vi "Update Mock Class.vi"(8 "error in (no error)":errorcluster, 10 "Mock Class Path":path=path "C:/Users/AntonSundqvist/Desktop/New folder/test.lvclass") -> (0 "error out":errorcluster)   [LabVIEW 2020, in "Mock Class Updater.lvclass"]
uses:
  Mock Class Updater.lvclass
  Mock Class Updater.lvclass/Mock Class Updater.ctl
  Mock Class Generator/Mock Class Generator.lvclass
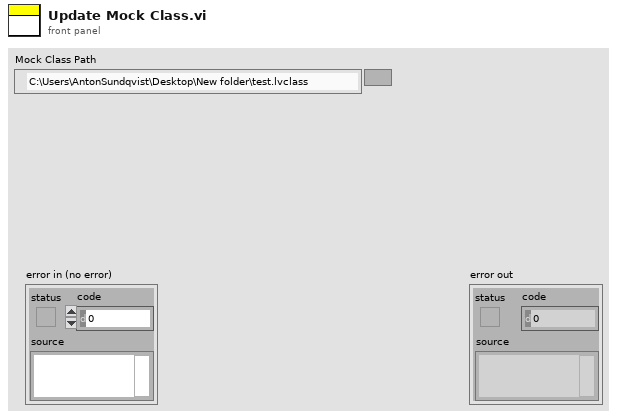
[diagram p1: front panel]
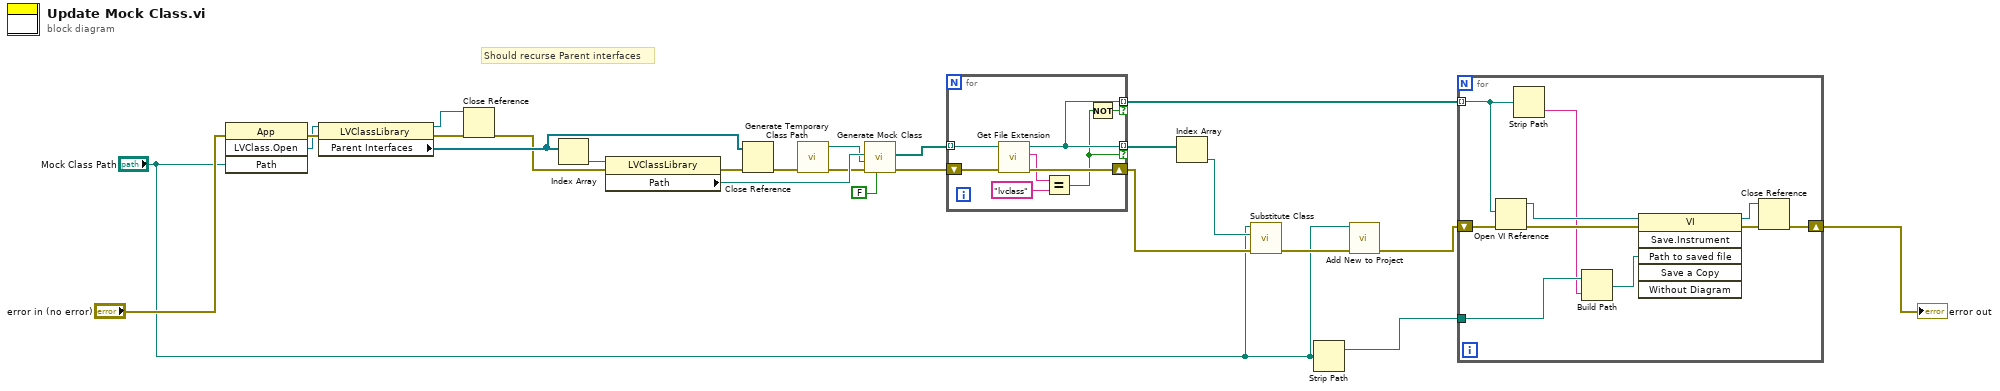
[diagram p0: block diagram]
diagram:
  # "Should recurse Parent interfaces"
  n1 = invoke class="App" method="LVClass.Open"(error in="error in (no error)", "Path"="Mock Class Path") -> (error out=w24:errorcluster, "LVClass.Open"=w23:refnum<vi>)  [unwired: 2 in, 2 out]
  n2 = property class="LVClassLibrary"(reference=w23, error in=w24) -> (reference out=w14:refnum<vi>, error out=w16:errorcluster, "Parent Interfaces"=w20:refnum<vi>[])
  n3 = Close Reference(reference=w14, error in (no error)=w16) -> (error out=w15:errorcluster)
  n4 = Index Array(array=w20) -> (element=w22:refnum<vi>)  [unwired: 1 in]
  n5 = property class="LVClassLibrary"(reference=w22, error in=w15) -> (error out=w21:errorcluster, "Path"=w19:path)  [unwired: 1 out]
  n6 = Close Reference(reference=w20, error in (no error)=w21) -> (error out=w18:errorcluster)
  n7 = call "Generate Temporary Class Path.vi"("error in (no error)"=w18) -> ("error out"=w5:errorcluster, "appended path"=w4:path)  [unwired: 9 in]
  n8 = call "Generate Mock Class.vi"("Add to lvproj?"=FALSE, "error in (no error)"=w5, "Destination Class Path"=w4, "Source Class Path"=w19) -> ("error out"=w12:errorcluster, "Created Files"=w13:path[])  [unwired: 6 in]
  n9 = for {
    tunnel: w13 -> [w33] mode=indexing
    shift-right: [w31] -> w11
    shift-left: w12 -> [w32]
    tunnel: [w28] -> w10 mode=indexing if=w27
    tunnel: [w28] -> w7 mode=indexing if=w26
    n10 = call <vilib>:"Get File Extension.vi"("error in (no error)"=w32, "file"=w33) -> ("error out"=w31:errorcluster, "lowercase file extension"=w30:string, "dup file"=w28:path)  [unwired: 5 in, 2 out]
    n11 = Equal?(x=w30, y="lvclass") -> (x = y?=w27:bool)
    n12 = Not(x=w27) -> (.not. x?=w26:bool)
  }
  n13 = Index Array(array=w10) -> (element=w2:path)  [unwired: 1 in]
  n14 = call "Substitute Class.vi"("error in (no error)"=w11, "New Class"=w2, "Class to Replace"="Mock Class Path") -> ("error out"=w9:errorcluster)  [unwired: 8 in]
  n15 = Strip Path(path="Mock Class Path") -> (stripped path=w6:path)  [unwired: 1 out]
  n16 = call "Add New to Project.vi"("error in (no error)"=w9, "Path"="Mock Class Path") -> ("error out"=w3:errorcluster)  [unwired: 9 in]
  n17 = for {
    shift-right: [w35] -> w8
    shift-left: w3 -> [w43]
    tunnel: w7 -> [w40] mode=indexing
    tunnel: w6 -> [w38]
    n18 = Open VI Reference(vi path=w40, error in (no error)=w43) -> (vi reference=w39:refnum<vi>, error out=w41:errorcluster)  [unwired: 4 in]
    n19 = Strip Path(path=w40) -> (name=w37:string)  [unwired: 1 out]
    n20 = Build Path(base path=w38, name or relative path=w37) -> (appended path=w36:path)
    n21 = invoke class="VI" method="Save.Instrument"(reference=w39, error in=w41, "Path to saved file"=w36) -> (reference out=w34:refnum<vi>, error out=w42:errorcluster)  [unwired: 3 in, 4 out]
    n22 = Close Reference(reference=w34, error in (no error)=w42) -> (error out=w35:errorcluster)
  }
  "error out" <- w8
